vi "PDF Protokoll HangUp.vi"(8 "error in (no error)":errorcluster caption="Fehler (Eingang, kein Fehler)") -> (0 "error out":errorcluster caption="Fehler (Ausgang)")   [LabVIEW 2020, in "Hangup Check.lvlib"]
uses:
  Hangup Check.lvlib
  AktionFGV Hangup.ctl
  Seiten/System Einstellungen V2/Aktioen FGV System Konstanten.ctl
  <vilib>/Utility/miscctls.llb/LVPrintingMarginsTypeDef.ctl
  Allgemein/allgemeine Sub-VIs.lvlib
  Seiten/System Einstellungen V2/System Einstellungen V2.lvlib
panel:
  out "Bestanden":bool caption="Boolesch"
  out "Grenzwert:":string
  out "Nullgas Messwert:":string
  out "Datenerfassungszeit:":string
  out "Nullgas Aufschaltzeit:":string
  out "Analysator:":string
  out "Aufschaltpunkt:":string
  out "Messbereich:":string
  out "Endzeit:":string
  out "Startzeit:":string
  out "Ser.Nr.:":string caption="Serien Nummer:"
  out "Messgerät:":string
  # "Hang - up Check"
  # "ppm"
  # "s"
  # "s"
  # "ppmC3"
  # "ppmC3"
  # "IAG-Industrie Automatisierungsgeschellschaft m.b.H.    l  Industriestraße 2    l    2722Weikersdorf     )+43262221734 7+43262221734655"
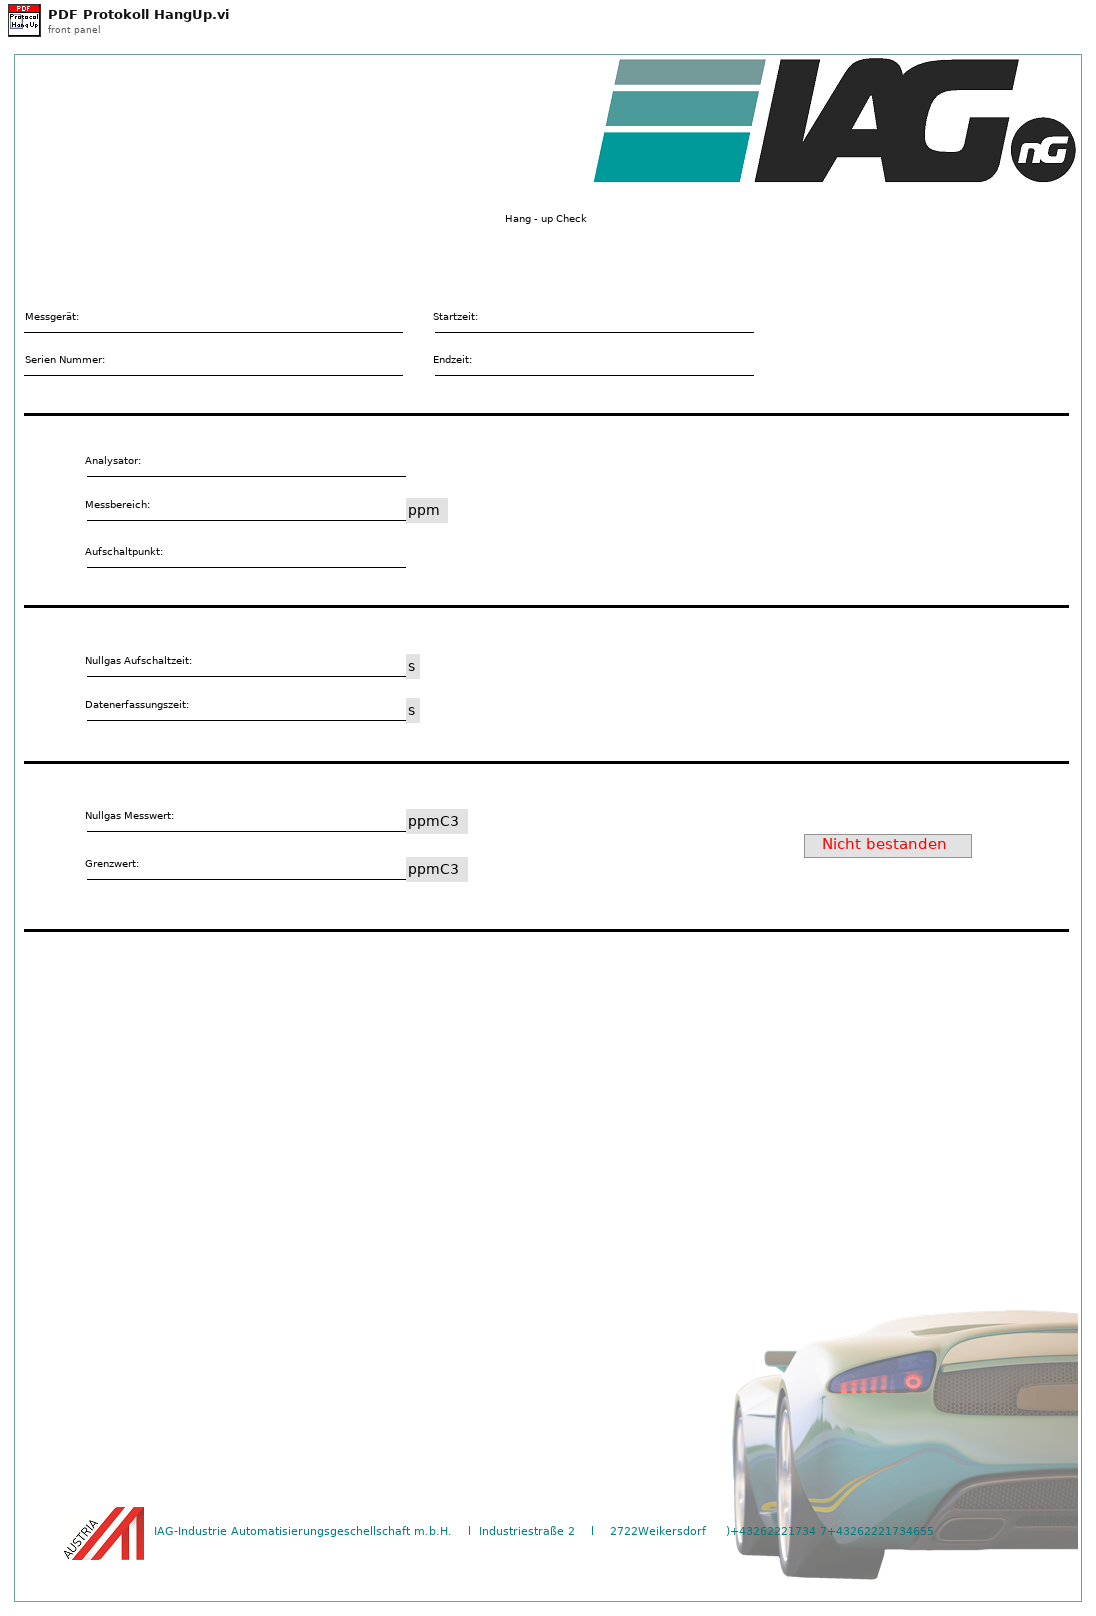
[diagram p1: front panel]
types:
  T1 = typedef "System Einstellungen V2.lvlib/Aktioen FGV System Konstanten.ctl" = enum16{"lesen", "laden", "speichern", "Sprache"}
  T2 = typedef "Hangup Check.lvlib/AktionFGV Hangup.ctl" = enum16{"lesen", "Hangup Settings", "Protokoll", "Pfad", "laden", "speichern"}
  T3 = enum32{"Portrait", "Landscape", "Rotated Portrait", "Rotated Landscape"}
  T4 = typedef "LVPrintingMarginsTypeDef.ctl" = cluster{"Top":sgl, "Left":sgl, "Bottom":sgl, "Right":sgl, "Measurement System":enum8{"Inches", "cm"}}
  T5 = typedef "Hangup Check.lvlib/HangupSettings.ctl" = cluster{"Kalibriergas":T6, "Aufschaltpunkt":T6, "Spangas Aufschaltzeit:":sgl, "Nullgas Aufschaltzeit:":sgl, "Datenerfassungszeit:":sgl, "Grenzwert manuell:":sgl, "Grenzwert:":sgl, "Grenze":T6, "Messbereich":T6, "Spankonzentration [ppm]":sgl, "Grenzwert: C1":sgl}
  T6 = typedef "Auswahlfeld.ctl" = u16
  T7 = typedef "Hangup Check.lvlib/Protokoll.ctl" = cluster{"FID Mittelwert 0":sgl, "FID Mittelwert E":sgl, "Messgasdruck Amium":sgl, "Startzeit":timestamp, "Endzeit":timestamp, "Bestanden?":bool}
  T8 = cluster{"Modell":string, "ProjektNummer":string, "Software Version":string, "Seriennummer":string}
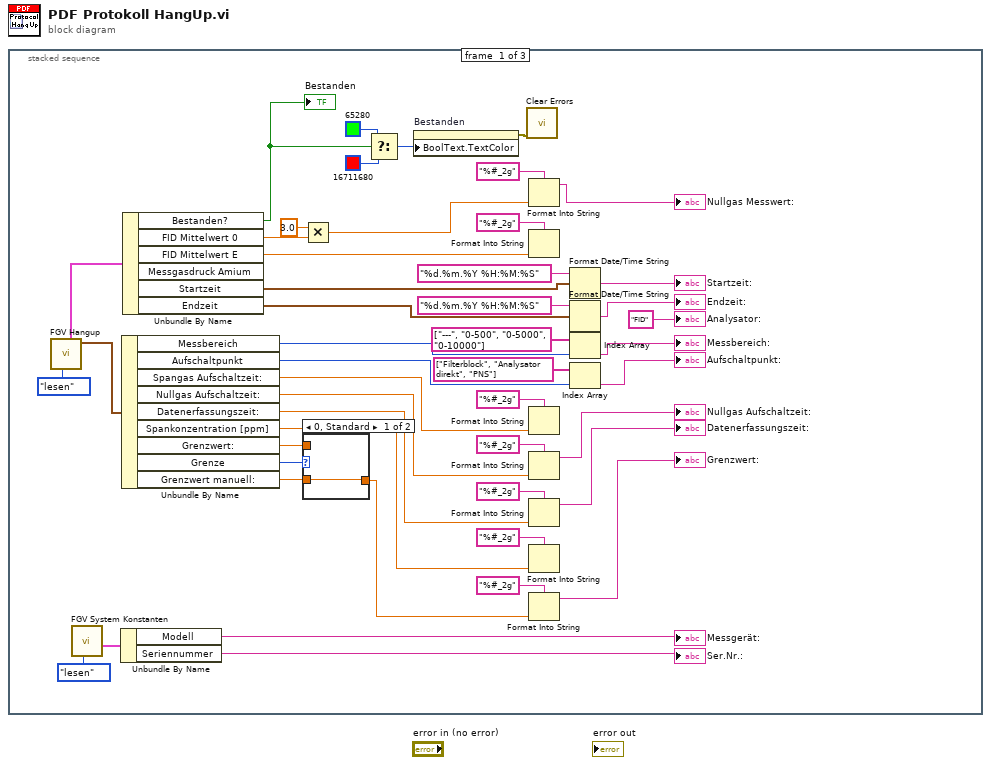
[diagram p0: block diagram]
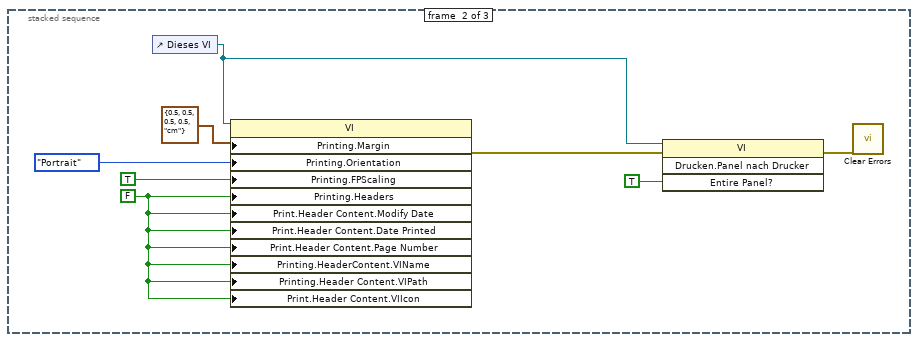
[diagram p3: hidden frame]
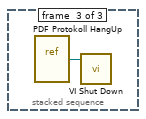
[diagram p4: hidden frame]
diagram:
  n1 = stacked-sequence {
    frame #0 {
      n2 = call "FGV Hangup.vi"("Aktion"=AktionFGV_Hangup."lesen") -> ("Hangup Settings"=w46:T5, "Protokoll"=w47:T7)  [unwired: 6 in, 3 out]
      n3 = call "FGV System Konstanten.vi"("Aktionen"=Aktioen_FGV_System_Konstanten."lesen") -> ("Cluster out"=w44:T8)  [unwired: 6 in, 4 out]
      n4 = Unbundle By Name(w44) -> ("Modell"=→"Messgerät:":string, "Seriennummer"=→"Ser.Nr.:":string)
      n5 = Unbundle By Name(w46) -> ("Messbereich"=w32:T6, "Aufschaltpunkt"=w31:T6, "Spangas Aufschaltzeit:"=w27:sgl, "Nullgas Aufschaltzeit:"=w25:sgl, "Datenerfassungszeit:"=w22:sgl, "Spankonzentration [ppm]"=w19:sgl, "Grenzwert:"=w16:sgl, "Grenze"=w18:T6, "Grenzwert manuell:"=w17:sgl)
      n6 = Unbundle By Name(w47) -> ("Bestanden?"=w1:bool, "FID Mittelwert 0"=w9:sgl, "FID Mittelwert E"=w11:sgl, "Startzeit"=w39:timestamp, "Endzeit"=w38:timestamp)  [unwired: 1 out]
      "Bestanden" <- w1
      n7 = Multiply(x=sgl 3.0 ("y"), y=w9) -> (x*y=w3:sgl)
      n8 = case shown="0, Standard" w18 {
        tunnel: w17 -> [w49 _]
        tunnel: [w49 w50] -> w15
        tunnel: w16 -> [_ w50]
        frame 0, Default {
        }
        frame 1 {
        }
      }
      n9 = Select(t=u32 65280, s=w1, f=u32 16711680) -> (s? t:f=w5:u32)
      n10 = property on="Bestanden" class="Bool. (strikt)"("BoolText.TextColor"=w5) -> (error out=w4:errorcluster)  [unwired: 2 in, 1 out]
      n11 = call <vilib>:"Clear Errors.vi"("error in (no error)"=w4) -> ()  [unwired: 5 in, 2 out]
      n12 = Format Into String(format string="%#_2g" ("Format-String"), w3) -> (resulting string=→"Nullgas Messwert:":string)  [unwired: 2 in, 1 out]
      n13 = Format Into String(format string="%#_2g" ("Format-String"), w11) -> ()  [unwired: 2 in, 2 out]
      n14 = Format Into String(format string="%#_2g" ("Format-String"), w27) -> ()  [unwired: 2 in, 2 out]
      n15 = Format Into String(format string="%#_2g" ("Format-String"), w25) -> (resulting string=→"Nullgas Aufschaltzeit:":string)  [unwired: 2 in, 1 out]
      n16 = Format Into String(format string="%#_2g" ("Format-String"), w22) -> (resulting string=→"Datenerfassungszeit:":string)  [unwired: 2 in, 1 out]
      n17 = Format Into String(format string="%#_2g" ("Format-String"), w19) -> ()  [unwired: 2 in, 2 out]
      n18 = Format Into String(format string="%#_2g" ("Format-String"), w15) -> (resulting string=→"Grenzwert:":string)  [unwired: 2 in, 1 out]
      n19 = Format Date/Time String(time format string (%c)="%d.%m.%Y %H:%M:%S" ("Zeitformatierungs-String (%c)"), seconds (now)=w39) -> (date/time string=→"Startzeit:":string)  [unwired: 1 in]
      n20 = Format Date/Time String(time format string (%c)="%d.%m.%Y %H:%M:%S" ("Zeitformatierungs-String (%c)"), seconds (now)=w38) -> (date/time string=→"Endzeit:":string)  [unwired: 1 in]
      n21 = Index Array(array=string[] ["---", "0-500", "0-5000", "0-10000"], index=w32) -> (element=→"Messbereich:":string)
      n22 = Index Array(array=string[] ["Filterblock", "Analysator direkt", "PNS"], index=w31) -> (element=→"Aufschaltpunkt:":string)
      "Analysator:" <- "FID" ("Analysator:")
    }
    frame #1 {
      w53 = FALSE ("Drucken:Kopfzeilen?")
      n23 = control-ref of="Dieses VI"() -> (w56:refnum<vi>)
      n24 = property class="VI"(reference=w56, "Printing.Margin"=T4 {"Top"=0.5, "Left"=0.5, "Bottom"=0.5, "Right"=0.5, "Measurement System"=enum."cm"} ("Drucken:Ränder"), "Printing.Orientation"=T3."Portrait" ("Drucken:Seitenausrichtung"), "Printing.FPScaling"=TRUE ("Drucken:Frontpanel-Skalierung?"), "Printing.Headers"=w53, "Print.Header Content.Modify Date"=w53, "Print.Header Content.Date Printed"=w53, "Print.Header Content.Page Number"=w53, "Printing.HeaderContent.VIName"=w53, "Printing.Header Content.VIPath"=w53, "Print.Header Content.VIIcon"=w53) -> (error out=w58:errorcluster)  [unwired: 1 in, 1 out]
      n25 = invoke class="VI" method="Drucken.Panel nach Drucker"(reference=w56, error in=w58, "Entire Panel?"=TRUE ("Abschnittskopfzeilen?")) -> (error out=w51:errorcluster)  [unwired: 1 in, 3 out]
      n26 = call <vilib>:"Clear Errors.vi"("error in (no error)"=w51) -> ()  [unwired: 5 in, 2 out]
    }
    frame #2 {
      n27 = vi-ref "PDF Protokoll HangUp.vi"() -> (w59:refnum<vi>)
      n28 = call "VI Shut Down.vi"("VI Referenz"=w59) -> ()  [unwired: 11 in]
    }
  }
